vi "iFlex Set Task.vi"(8 "error in (no error)":errorcluster, 11 "params":variant=variant(cluster{"New LSM Settings":cluster{"Multi Frame Count":dbl, "Trigger Mode":dbl, "Channel Selection":enum32{"A", "B", "AB"}, "Pixel Count":cluster{"Pixels in X":u32, "Pixels in Y":u32}, "Field Size":dbl, "Area Mode":dbl, "Frames":u8, "Averaging":bool, "Alignment":dbl, "Scan Mode":bool, "Gain":cluster{"Gain A":u8, "Gain B":u8}, "Enable PMTs":cluster{"A":bool, "B":bool}, "Voltage Range":cluster{"Range A":u16, "Range B":u16}, "Real Time Averaging":bool, "PFOV":dbl, "MicronsPerPx":dbl}, "index of element":i32} {"New LSM Settings"={"Multi Frame Count"=0.0, "Trigger Mode"=2.0, "Channel Selection"=enum."A", "Pixel Count"={"Pixels in X"=32, "Pixels in Y"=32}, "Field Size"=90.0, "Area Mode"=1.0, "Frames"=2, "Averaging"=FALSE, "Alignment"=0.0, "Scan Mode"=TRUE, "Gain"={"Gain A"=1, "Gain B"=1}, "Enable PMTs"={"A"=TRUE, "B"=TRUE}, "Voltage Range"={"Range A"=10, "Range B"=10}, "Real Time Averaging"=TRUE, "PFOV"=0.0, "MicronsPerPx"=0.0}, "index of element"=13})) -> (0 "error out":errorcluster, 3 "iFlex Control out":T1)   [LabVIEW 2020]
uses:
  <vilib>/DAQmx/write.llb/DAQmx Write (Digital Bool 1Line 1Point).vi
  <vilib>/DAQmx/write.llb/DAQmx Write (Analog DBL 1Chan 1Samp).vi
  <vilib>/DAQmx/miscellaneous.llb/DAQmx Fill In Error Info.vi
panel:
  in  "iFlex Control in":T1
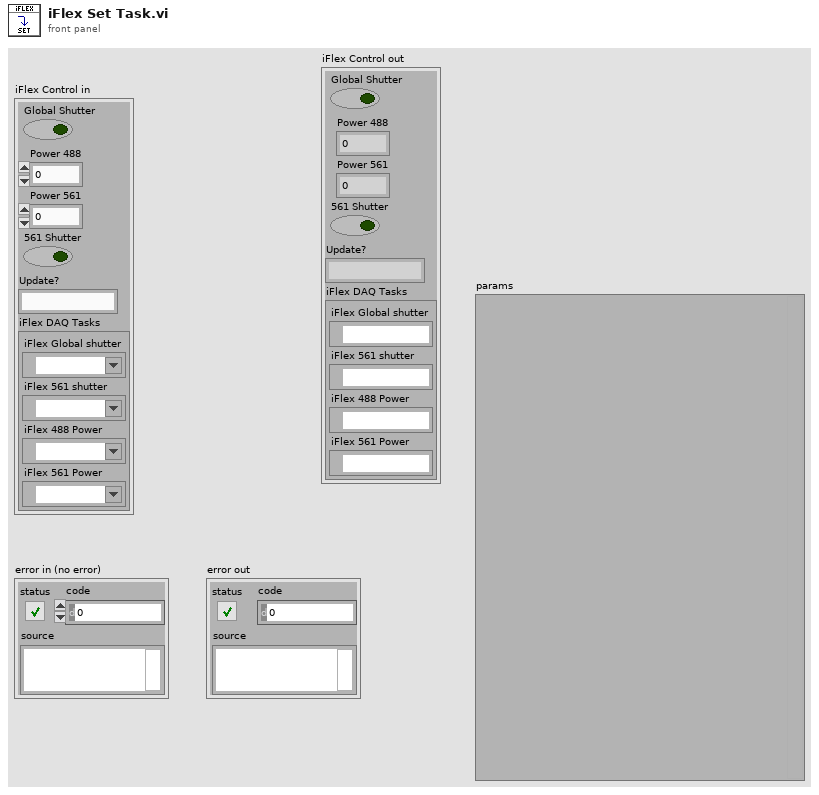
[diagram p1: front panel]
types:
  T1 = cluster{"Global Shutter":bool, "Power 488":dbl, "Power 561":dbl, "561 Shutter":bool, "Update?":string, "iFlex DAQ Tasks":cluster{"iFlex Global shutter":refnum<k21>, "iFlex 561 shutter":refnum<k21>, "iFlex 488 Power":refnum<k21>, "iFlex 561 Power":refnum<k21>}}
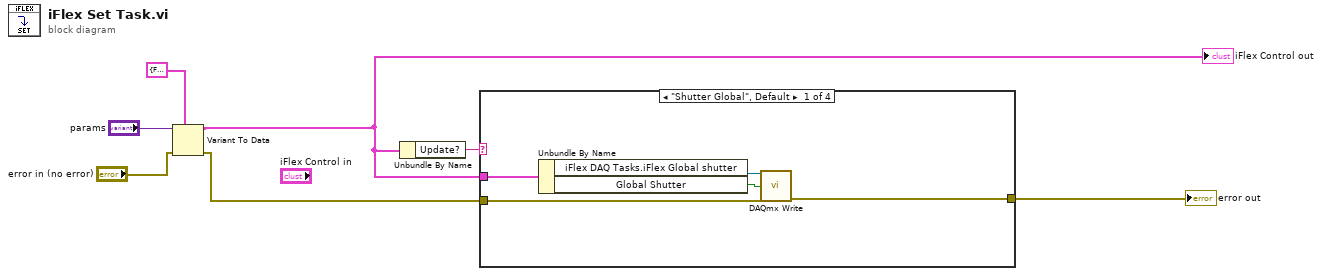
[diagram p0: block diagram]
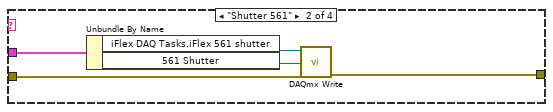
[diagram p2: hidden frame]
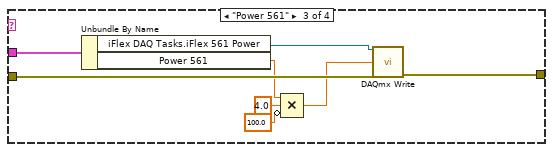
[diagram p3: hidden frame]
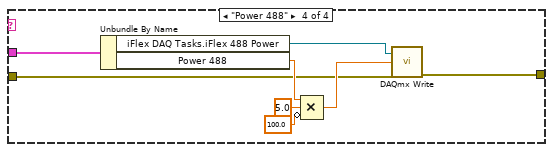
[diagram p4: hidden frame]
diagram:
  n1 = Variant To Data(error in="error in (no error)", type=T1 {"Global Shutter"=FALSE, "Power 488"=0.0, "Power 561"=0.0, "561 Shutter"=FALSE, "Update?"="", "iFlex DAQ Tasks"={"iFlex Global shutter"="", "iFlex 561 shutter"="", "iFlex 488 Power"="", "iFlex 561 Power"=""}} ("NewVal"), Variant="params") -> (data=w3:T1, error out=w1:errorcluster)
  "iFlex Control out" <- w3
  n2 = Unbundle By Name(w3) -> ("Update?"=w7:string)
  n3 = case shown="\"Shutter Global\", Default" w7 {
    tunnel: w3 -> [w12 w15 w18 w26]
    tunnel: w1 -> [w9 w14 w24 w27]
    tunnel: [w8 w13 w25 w28] -> w6
    frame "Shutter Global", Default {
      n4 = Unbundle By Name(w12) -> ("iFlex DAQ Tasks.iFlex Global shutter"=w11:refnum<k21>, "Global Shutter"=w10:bool)
      n5 = call-poly <vilib>:"DAQmx Write.vi"("task/channels in"=w11, "data"=w10, "error in"=w9) -> ("error out"=w8:errorcluster)  [unwired: 10 in, 2 out]
    }
    frame "Shutter 561" {
      n6 = Unbundle By Name(w15) -> ("iFlex DAQ Tasks.iFlex 561 shutter"=w17:refnum<k21>, "561 Shutter"=w16:bool)
      n7 = call-poly <vilib>:"DAQmx Write.vi"("task/channels in"=w17, "data"=w16, "error in"=w14) -> ("error out"=w13:errorcluster)  [unwired: 10 in, 2 out]
    }
    frame "Power 561" {
      n8 = Unbundle By Name(w18) -> ("iFlex DAQ Tasks.iFlex 561 Power"=w23:refnum<k21>, "Power 561"=w20:dbl)
      n9 = Compound Arithmetic op=MULTIPLY(w20, 4.0 ("value"), invert 100.0 ("y")) -> (w19:dbl)
      n10 = call-poly <vilib>:"DAQmx Write.vi"("task/channels in"=w23, "data"=w19, "error in"=w24) -> ("error out"=w25:errorcluster)  [unwired: 10 in, 2 out]
    }
    frame "Power 488" {
      n11 = Unbundle By Name(w26) -> ("iFlex DAQ Tasks.iFlex 488 Power"=w33:refnum<k21>, "Power 488"=w30:dbl)
      n12 = Compound Arithmetic op=MULTIPLY(w30, 5.0 ("value"), invert 100.0 ("y")) -> (w29:dbl)
      n13 = call-poly <vilib>:"DAQmx Write.vi"("task/channels in"=w33, "data"=w29, "error in"=w27) -> ("error out"=w28:errorcluster)  [unwired: 10 in, 2 out]
    }
  }
  "error out" <- w6
